vi "Camera handle.vi"(0 "axis 2 (y)":dbl, 1 "axis 3 (rotation)":dbl, 2 "Center on Target":bool, 3 "View Ground":bool, 7 "Stop Auto Cam movement":bool, 8 "Camera X axis center angle":i32, 9 "Seen floor angle Y":i32, 10 "Servo Get Angle X":i32, 11 "Servo Get Angle Y":i32) -> (16 "Out X [angle]":i32, 17 "Out Y [angle]":i32, 19 "Camera Centered on Target":bool)   [LabVIEW 2012]
uses:
  BotStatus.vi
panel:
  # "Angle"
  # "Angle"
  # "Angle"
  # "Angle"
  # "Valid for 3Dpro joystick\nif another joystick is used use the Y axis"
  # "Angle"
  # "Angle"
  # "Angle"
  # "Angle"
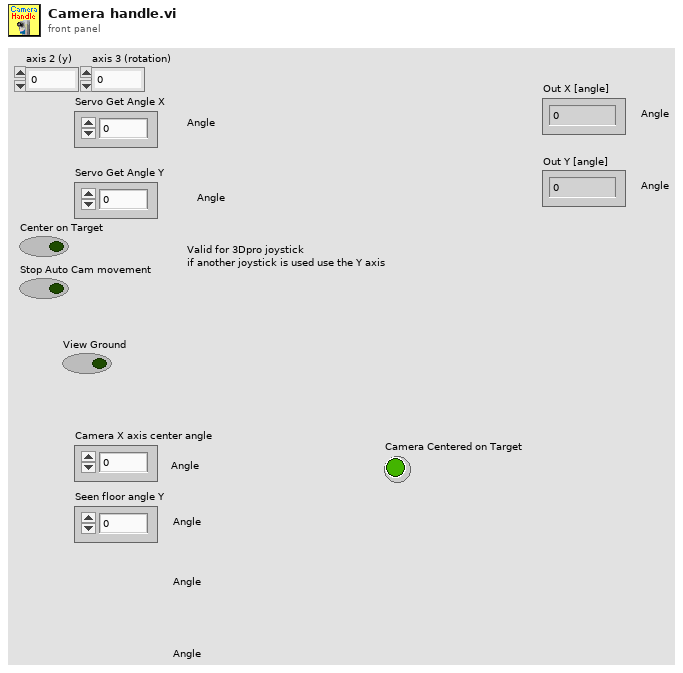
[diagram p1: front panel]
types:
  T1 = cluster{"Target Position X":dbl, "Target Position Y":dbl, "Target Found":bool}
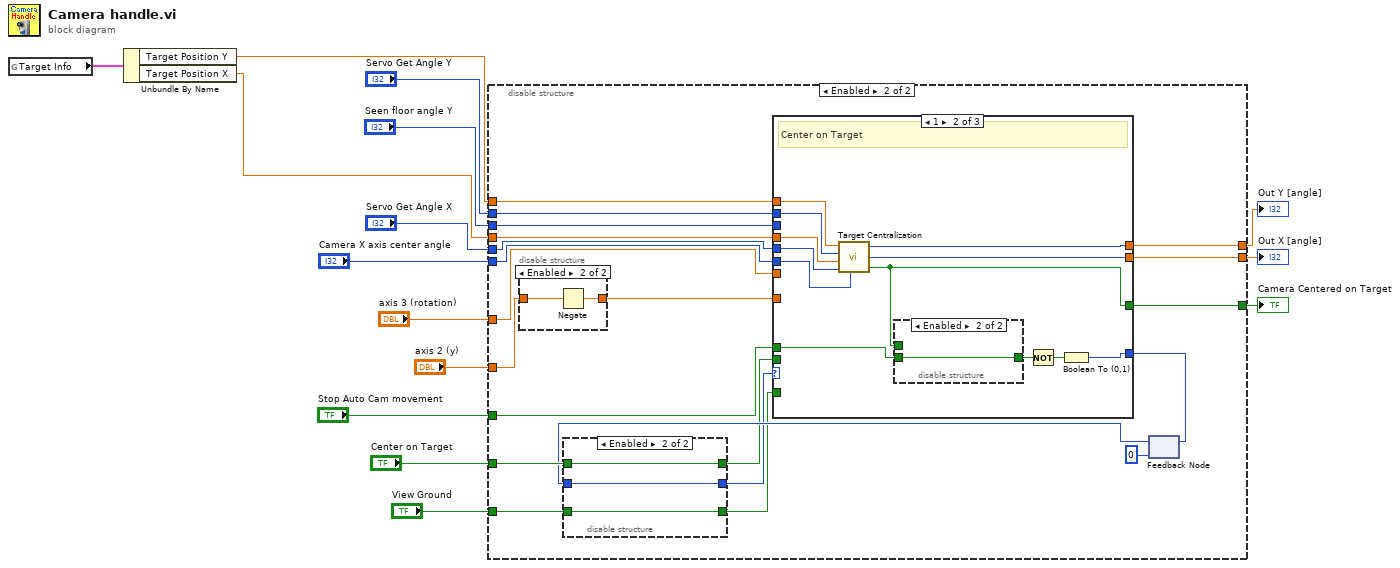
[diagram p0: block diagram]
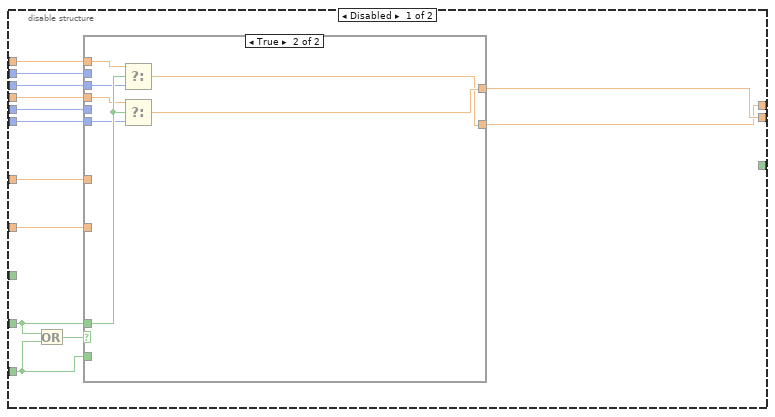
[diagram p2: hidden frame]
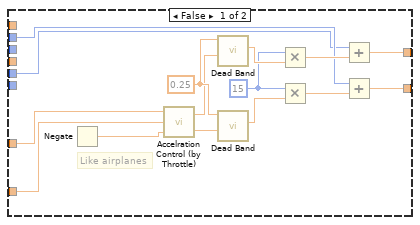
[diagram p3: hidden frame]
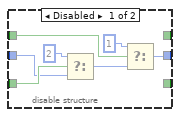
[diagram p4: hidden frame]
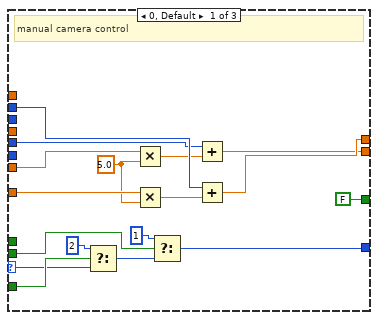
[diagram p6: hidden frame]
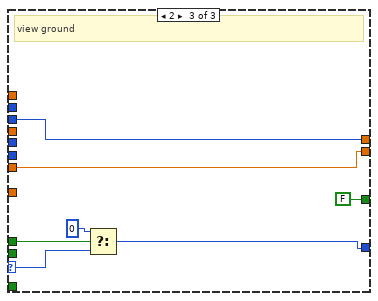
[diagram p8: hidden frame]
diagram:
  n1 = global read "BotStatus.vi" "Target Info"() -> (w3:T1)
  n2 = Unbundle By Name(w3) -> ("Target Position Y"=w2:dbl, "Target Position X"=w1:dbl)
  n3 = disable-structure shown="Enabled" {
    disable-tunnel: [w28 w70] -> w15
    disable-tunnel: [w27 w68] -> w14
    disable-tunnel: "Servo Get Angle X" -> [w26 w63]
    disable-tunnel: "Servo Get Angle Y" -> [w25 w65]
    disable-tunnel: "axis 3 (rotation)" -> [w23 w64]
    disable-tunnel: "axis 2 (y)" -> [w22 w66]
    disable-tunnel: "Center on Target" -> [w21 w56]
    disable-tunnel: "View Ground" -> [w20 w55]
    disable-tunnel: "Seen floor angle Y" -> [w19 w69]
    disable-tunnel: "Camera X axis center angle" -> [w18 w71]
    disable-tunnel: w1 -> [w17 w61]
    disable-tunnel: w2 -> [w16 w62]
    disable-tunnel: [_ w60] -> w9
    disable-tunnel: "Stop Auto Cam movement" -> [_ w58]
    frame Disabled {
      n4 = Or(x=w21, y=w20) -> (x .or. y?=w24:bool)
      n5 = case shown="True" w24 {
        tunnel: [w31 w50] -> w28
        tunnel: [w30 w49] -> w27
        tunnel: w26 -> [w37 _]
        tunnel: w25 -> [w38 _]
        tunnel: w23 -> [w33 _]
        tunnel: w22 -> [w32 _]
        tunnel: w21 -> [_ w48]
        tunnel: w20 -> [_ _]
        tunnel: w19 -> [_ w47]
        tunnel: w18 -> [_ w46]
        tunnel: w17 -> [_ w45]
        tunnel: w16 -> [_ w44]
        frame False {
          w36 = 15
          w43 = 0.25 ("Dead Band")
          # "Like airplanes"
          n6 = Negate() -> (-x=w29:dbl)  [unwired: 1 in]
          n7 = call "Accelration Control (by Throttle).vi"("acc"=w29, "Yinput"=w32, "Xinput"=w33) -> ("Youtput"=w34:dbl, "Xoutput"=w35:dbl)
          n8 = call "Dead Band.vi"("Axis In"=w35, "Dead Band"=w43) -> ("Axis Out"=w42:dbl)  [unwired: 9 in]
          n9 = call "Dead Band.vi"("Axis In"=w34, "Dead Band"=w43) -> ("Axis Out"=w41:dbl)  [unwired: 9 in]
          n10 = Multiply(x=w36, y=w42) -> (x*y=w39:dbl)
          n11 = Multiply(x=w36, y=w41) -> (x*y=w40:dbl)
          n12 = Add(x=w37, y=w39) -> (x+y=w31:dbl)
          n13 = Add(x=w38, y=w40) -> (x+y=w30:dbl)
        }
        frame True {
          n14 = Select(t=w44, s=w48, f=w47) -> (s? t:f=w49:dbl)
          n15 = Select(t=w45, s=w48, f=w46) -> (s? t:f=w50:dbl)
        }
      }
    }
    frame Enabled {
      n16 = disable-structure shown="Enabled" {
        disable-tunnel: [w82 w83] -> w67
        disable-tunnel: w66 -> [w82 w84]
        frame Disabled {
        }
        frame Enabled {
          n17 = Negate(x=w84) -> (-x=w83:dbl)
        }
      }
      n18 = feedback #1(i16 0) -> (w54:i16)
      n19 = disable-structure shown="Enabled" {
        disable-tunnel: w56 -> [w78 w80]
        disable-tunnel: w55 -> [w76 w79]
        disable-tunnel: w54 -> [w74 w81]
        disable-tunnel: [w72 w81] -> w53
        disable-tunnel: [_ w80] -> w52
        disable-tunnel: [_ w79] -> w51
        frame Disabled {
          n20 = Select(t=i16 2, s=w76, f=w74) -> (s? t:f=w73:i16)
          n21 = Select(t=i16 1, s=w78, f=w73) -> (s? t:f=w72:i16)
        }
        frame Enabled {
        }
      }
      n22 = case shown="1" w53 {
        selector: w53 -> [w86 _ w117]
        tunnel: w71 -> [_ w109 _]
        tunnel: [w92 w107 w122] -> w70
        tunnel: w69 -> [_ _ w120]
        tunnel: [w93 w108 w120] -> w68
        tunnel: w67 -> [w101 _ _]
        tunnel: w65 -> [w99 w112 _]
        tunnel: w64 -> [w97 _ w122]
        tunnel: w63 -> [w96 w110 _]
        tunnel: w62 -> [_ w113 _]
        tunnel: w61 -> [_ w111 _]
        tunnel: [FALSE ("centered") w104 FALSE ("centered")] -> w60
        tunnel: [w85 w105 w116] -> w59
        tunnel: w58 -> [_ w102 w119]
        tunnel: w52 -> [w88 _ _]
        tunnel: w51 -> [w87 _ _]
        frame 0, Default {
          w95 = 5.0 ("y")
          # "manual camera control"
          n23 = Select(t=i16 2, s=w87, f=w86) -> (s? t:f=w91:i16)
          n24 = Multiply(x=w97, y=w95) -> (x*y=w98:dbl)
          n25 = Multiply(x=w101, y=w95) -> (x*y=w100:dbl)
          n26 = Select(t=i16 1, s=w88, f=w91) -> (s? t:f=w85:i16)
          n27 = Add(x=w96, y=w98) -> (x+y=w92:dbl)
          n28 = Add(x=w99, y=w100) -> (x+y=w93:dbl)
        }
        frame 1 {
          # "Center on Target"
          n29 = call "Target Centralization.vi"("Target Position Y"=w113, "Servo Get Angle Y"=w112, "Target Position X"=w111, "X axis center angle"=w109, "Servo Get Angle X"=w110) -> ("Servo Angle Set Point Y"=w108:i32, "Servo Angle Set Point X"=w107:i32, "centered"=w104:bool)  [unwired: 1 in]
          n30 = disable-structure shown="Enabled" {
            disable-tunnel: [w114 w115] -> w103
            disable-tunnel: w104 -> [w114 _]
            disable-tunnel: w102 -> [_ w115]
            frame Disabled {
            }
            frame Enabled {
            }
          }
          n31 = Not(x=w103) -> (.not. x?=w106:bool)
          n32 = Boolean To (0,1)(Boolean=w106) -> (0, 1=w105:i16)
        }
        frame 2 {
          # "view ground"
          n33 = Select(t=i16 0, s=w119, f=w117) -> (s? t:f=w116:i16)
        }
      }
      n34 = feedback-in #1(w59) -> ()
    }
  }
  "Out X [angle]" <- w15
  "Out Y [angle]" <- w14
  "Camera Centered on Target" <- w9
